vi "GetDataGroupChannels.vi"(8 "error in (no error)":errorcluster, 9 "group":string, 10 "923x acquisition config":T1 {"FixedSizeX31"."InputConfig" items=["AC Coupled", "DC Coupled", "IEPE AC Coupled"]}, 11 "all waveforms":waveform(sgl)[](array[waveform])) -> (0 "error out":errorcluster, 3 "this groups channels":waveform(sgl)[](array[waveform]))   [LabVIEW 2017, in "McsaFpgaAcquisition.lvlib"]
uses:
  <vilib>/addons/InsightCM/Devices/Shared/Mcsa/McsaFpgaAcquisition/McsaFpgaAcquisition.lvlib
  <vilib>/addons/InsightCM/Devices/Shared/Mcsa/McsaFpgaAcquisition/controls/Configuration.ctl
  <vilib>/addons/InsightCM/Devices/Shared/Cms/CmsAcquisition/controls/FixedSizeArrays.ctl
  <vilib>/LabVIEW Targets/FPGA/cRIO/shared/nicrio_ModuleControls/nicrio_cRIO-9232_ConfigModeRing.ctl
  <vilib>/addons/InsightCM/Devices/Shared/Cms/cRIOWfmAcq/subVIs/RIO Wfm Cust Ctrls/rwfm_SamplingInfo.ctl
  <vilib>/addons/InsightCM/Devices/Shared/Mcsa/McsaFpgaAcquisition/controls/Group.ctl
  <vilib>/addons/InsightCM/Devices/Shared/Mcsa/McsaFpgaAcquisition/controls/ChannelMcsa.ctl
  <vilib>/addons/InsightCM/Devices/Shared/Mcsa/McsaFpgaAcquisition/controls/RangeParams.ctl
  <vilib>/addons/InsightCM/Devices/Shared/Cms/cRIOWfmAcq/cRIOWfmLib.lvlib
  <vilib>/addons/InsightCM/Devices/Shared/Cms/CmsAcquisition/CmsAcquisition.lvlib
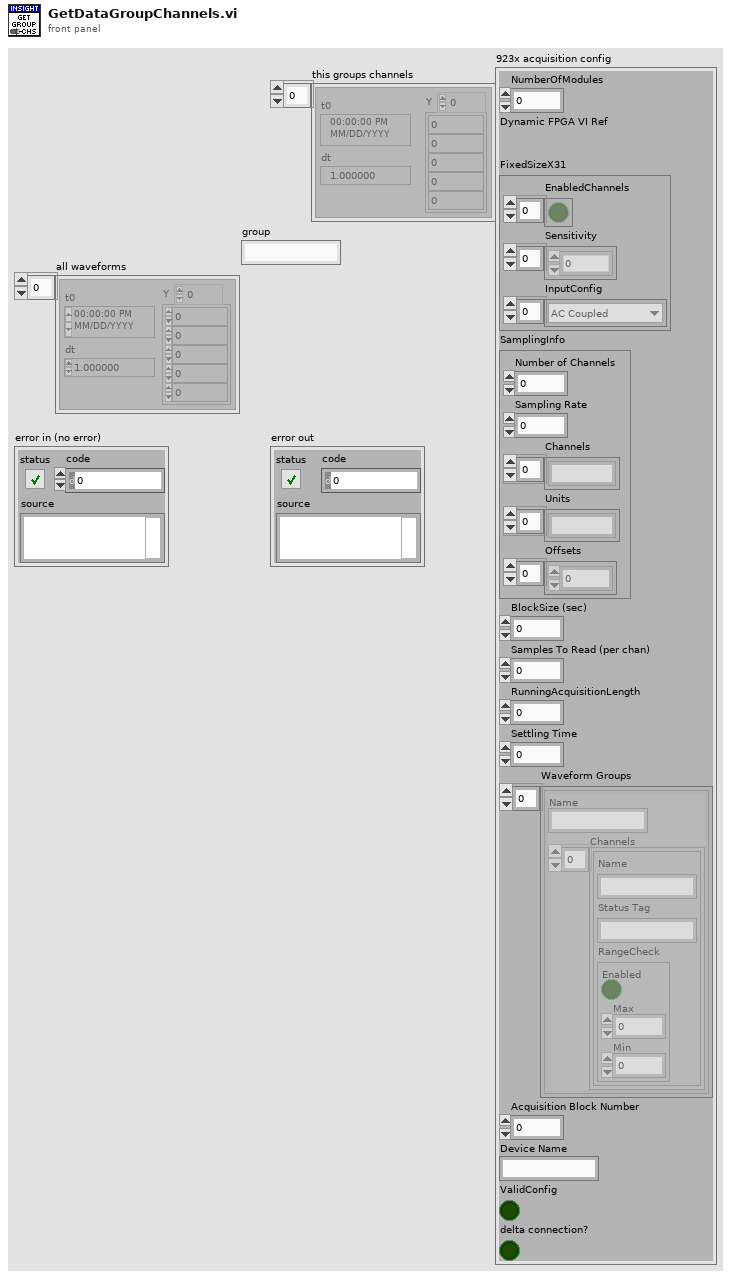
[diagram p1: front panel]
types:
  T1 = typedef "McsaFpgaAcquisition.lvlib/Configuration.ctl" = cluster{"NumberOfModules":i16, "Dynamic FPGA VI Ref":refnum<k20>, "FixedSizeX31":T2, "SamplingInfo":T4, "BlockSize (sec)":dbl, "Samples To Read (per chan)":i32, "RunningAcquisitionLength":dbl, "Settling Time":dbl, "Waveform Groups":T5[], "Acquisition Block Number":i32, "Device Name":string, "ValidConfig":bool, "delta connection?":bool}
  T2 = typedef "CmsAcquisition.lvlib/FixedSizeArrays.ctl" = cluster{"EnabledChannels":bool[], "Sensitivity":dbl[], "InputConfig":T3[]}
  T3 = typedef "nicrio_cRIO-9232_ConfigModeRing.ctl" = u8
  T4 = typedef "cRIOWfmLib.lvlib/rwfm_SamplingInfo.ctl" = cluster{"Number of Channels":i32, "Sampling Rate":dbl, "Channels":string[], "Units":string[], "Offsets":sgl[]}
  T5 = typedef "McsaFpgaAcquisition.lvlib/Group.ctl" = cluster{"Name":string, "Channels":T6[]}
  T6 = typedef "McsaFpgaAcquisition.lvlib/ChannelMcsa.ctl" = cluster{"Name":string, "Status Tag":string, "RangeCheck":T7}
  T7 = typedef "McsaFpgaAcquisition.lvlib/RangeParams.ctl" = cluster{"Enabled":bool, "Max":dbl, "Min":dbl}
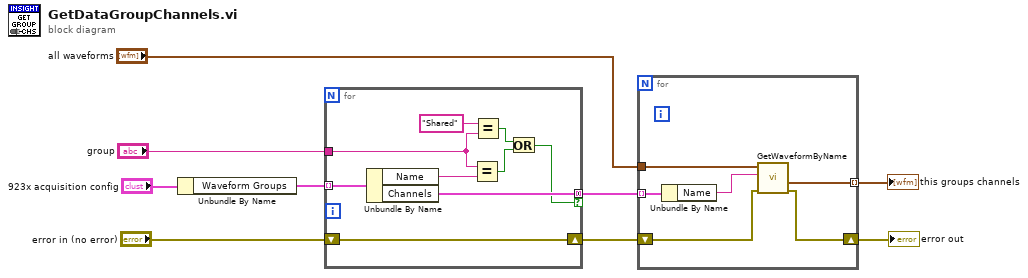
[diagram p0: block diagram]
diagram:
  n1 = Unbundle By Name("923x acquisition config") -> ("Waveform Groups"=w5:T5[])
  n2 = for {
    shift-right: [w18] -> w2
    shift-left: "error in (no error)" -> [w18]
    tunnel: w5 -> [w17] mode=indexing
    tunnel: "group" -> [w15]
    tunnel: [w11] -> w3 mode=concatenating if=w10
    n3 = Unbundle By Name(w17) -> ("Name"=w16:string, "Channels"=w11:T6[])
    n4 = Equal?(x=w15, y=w16) -> (x = y?=w13:bool)
    n5 = Equal?(x="Shared", y=w15) -> (x = y?=w12:bool)
    n6 = Or(x=w12, y=w13) -> (x .or. y?=w10:bool)
  }
  n7 = for {
    tunnel: "all waveforms" -> [w24]
    shift-right: [w22] -> w8
    shift-left: w2 -> [w23]
    tunnel: [w21] -> w1 mode=indexing
    tunnel: w3 -> [w20] mode=indexing
    n8 = Unbundle By Name(w20) -> ("Name"=w19:string)
    n9 = call <vilib>:"GetWaveformByName.vi"("error in (no error)"=w23, "Channel Name"=w19, "Acq Waveforms"=w24) -> ("error out"=w22:errorcluster, "Waveform"=w21:waveform(sgl))  [unwired: 5 in, 2 out]
  }
  "this groups channels" <- w1
  "error out" <- w8
